vi "Data_Logger.vi"(3 "Salvar Dados":bool, 5 "Sobrescrever arquivo ?":bool=TRUE, 6 "Constante de Calibração":dbl, 7 "Diretório\nh":path, 8 "stop 2":bool, 9 "Sinal do Gerador":tag, 10 "Contador":tag="/Dev1/PFI7", 11 "Entrada do Sinal":tag) -> ()   [LabVIEW 2025]
uses:
  <vilib>/DAQmx/read.llb/DAQmx Read (Analog Wfm 1Chan NSamp).vi
  <vilib>/DAQmx/read.llb/DAQmx Read (Counter U32 1Chan 1Samp).vi
  <resource>/objmgr/daqmx.rc
  <vilib>/Waveform/WDTFileIO.llb/Export Waveform To Spreadsheet File.vi
  <vilib>/DAQmx/create/channels.llb/DAQmx Create Channel (AI-Voltage-Basic).vi
  <vilib>/DAQmx/configure/timing.llb/DAQmx Timing (Sample Clock).vi
  <vilib>/DAQmx/create/channels.llb/DAQmx Create Channel (CI-Count Edges).vi
panel:
  in  "Tab Control":T1(tab)
  out "Waveform Graph":waveform(dbl)(graph)
  out "Loop Count":i32
  out "Distância (mm)":u32
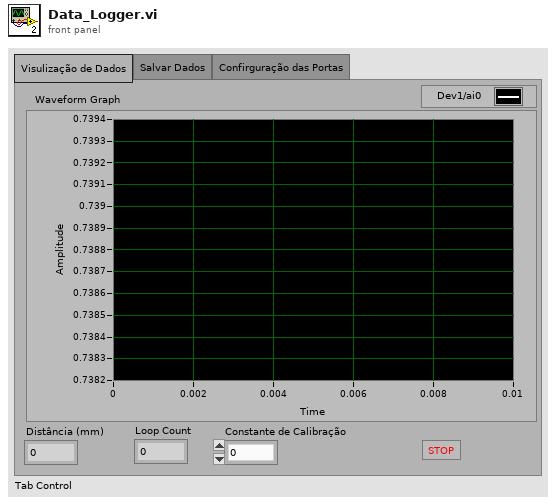
[diagram p1: front panel]
types:
  T1 = enum32{"Visulização de Dados", "Salvar Dados", "Confirguração das Portas"}
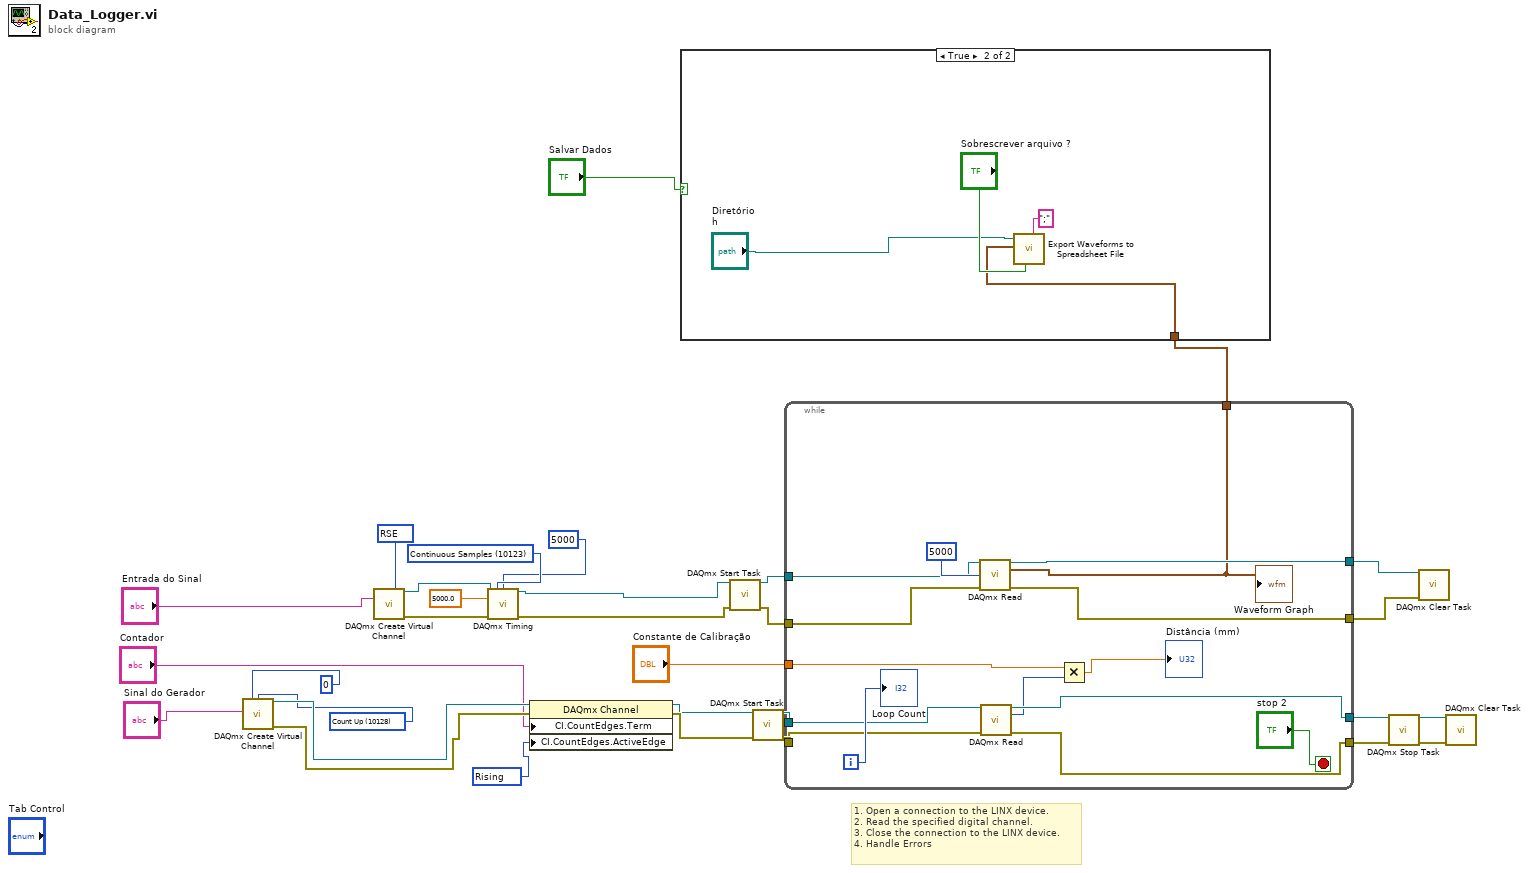
[diagram p0: block diagram]
diagram:
  w13 = 10280 items=["Rising"=10280, "Falling"=10171] ("CI.CountEdges.ActiveEdge")
  w11 = 10128 items=["Count Up"=10128, "Count Down"=10124, "Externally Controlled"=10326] ("count direction")
  w7 = 10083 items=["Default"=-1, "RSE"=10083, "NRSE"=10078, "Differential"=10106, "Pseudodifferential"=12529] ("input terminal configuration")
  w10 = 10123 items=["Finite Samples"=10178, "Continuous Samples"=10123, "Hardware Timed Single Point"=12522] ("sample mode")
  # "1. Open a connection to the LINX device.\n2. Read the specified digital channel.\n3. Close the connection to the LINX device.\n4. Handle Errors"
  n1 = call-poly <vilib>:"DAQmx Create Virtual Channel.vi"("initial count"=u32 0, "count direction"=w11, "counter"="Sinal do Gerador") -> ("task out"=w22:refnum<k21>, "error out"=w23:errorcluster)  [unwired: 11 in]
  n2 = call-poly <vilib>:"DAQmx Create Virtual Channel.vi"("input terminal configuration"=w7, "physical channels"="Entrada do Sinal") -> ("task out"=w15:refnum<k21>, "error out"=w16:errorcluster)  [unwired: 12 in]
  n3 = call-poly <vilib>:"DAQmx Timing.vi"("task/channels in"=w15, "sample mode"=w10, "samples per channel"=5000, "rate"=5000.0, "error in"=w16) -> ("task out"=w20:refnum<k21>, "error out"=w21:errorcluster)  [unwired: 9 in]
  n4 = property class="DAQmx Channel"(reference=w22, error in=w23, "CI.CountEdges.Term"="Contador", "CI.CountEdges.ActiveEdge"=w13) -> (reference out=w24:refnum<k21>, error out=w25:errorcluster)
  n5 = call <vilib>:"DAQmx Start Task.vi"("task/channels in"=w20, "error in"=w21) -> ("task out"=w18:refnum<k21>, "error out"=w19:errorcluster)  [unwired: 12 in]
  n6 = call <vilib>:"DAQmx Start Task.vi"("task/channels in"=w24, "error in"=w25) -> ("task out"=w26:refnum<k21>, "error out"=w27:errorcluster)  [unwired: 12 in]
  n7 = while {
    tunnel: [w45] -> w17
    tunnel: [w46] -> w14
    tunnel: w18 -> [w41]
    tunnel: w19 -> [w40]
    tunnel: w26 -> [w39]
    tunnel: w27 -> [w38]
    tunnel: [w37] -> w30
    tunnel: [w36] -> w31
    tunnel: [w33] -> w5
    tunnel: "Constante de Calibração" -> [w32]
    i -> [w42]
    stop <- "stop 2" stop-if-true
    n8 = call-poly <vilib>:"DAQmx Read.vi"("task/channels in"=w41, "number of samples per channel"=5000, "error in"=w40) -> ("task out"=w46:refnum<k21>, "data"=w33:waveform(dbl), "error out"=w45:errorcluster)  [unwired: 10 in]
    "Waveform Graph" <- w33
    n9 = call-poly <vilib>:"DAQmx Read.vi"("task/channels in"=w39, "error in"=w38) -> ("task out"=w37:refnum<k21>, "data"=w35:u32, "error out"=w36:errorcluster)  [unwired: 11 in]
    n10 = Multiply(x=w32, y=w35) -> (x*y=→"Distância (mm)":dbl)
    "Loop Count" <- w42
  }
  n11 = case shown="True" "Salvar Dados" {
    tunnel: w5 -> [_ w47]
    frame False {
    }
    frame True {
      n12 = call-poly <vilib>:"Export Waveforms to Spreadsheet File.vi"("delimiter (Tab)"=";", "append to file? (new file:F)"="Sobrescrever arquivo ?", "waveform"=w47, "file path (dialog if empty)"="Diretório\nh") -> ()  [unwired: 6 in, 2 out]
    }
  }
  n13 = call <vilib>:"DAQmx Stop Task.vi"("task/channels in"=w30, "error in"=w31) -> ("task out"=w28:refnum<k21>, "error out"=w29:errorcluster)  [unwired: 12 in]
  n14 = call <vilib>:"DAQmx Clear Task.vi"("task in"=w14, "error in"=w17) -> ()  [unwired: 13 in, 1 out]
  n15 = call <vilib>:"DAQmx Clear Task.vi"("task in"=w28, "error in"=w29) -> ()  [unwired: 13 in, 1 out]
